vi "RTM Add a new channel.vi"(8 "error in (no error)":errorcluster, 11 "Node Ptr":u64 format="%.0x") -> (0 "error out":errorcluster)   [LabVIEW 2016, in "Async UDP System Explorer.lvlib"]
uses:
  System Explorer/Async UDP System Explorer.lvlib
  <vilib>/NI Veristand/Custom Device API/Custom Device Channel.ctl
  <vilib>/NI Veristand/Custom Device API/Custom Device Channel Type.ctl
  <vilib>/NI Veristand/Custom Device API/Custom Device API.lvlib
panel:
  in  "Tag":string
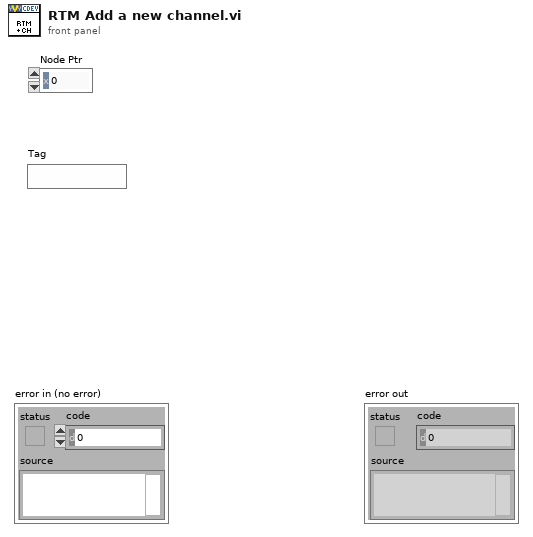
[diagram p1: front panel]
types:
  T1 = typedef "Custom Device API.lvlib/Custom Device Channel.ctl" = cluster{"Type":T2, "Units":string, "Default Value":dbl, "Faultable":bool, "Scalable":bool}
  T2 = typedef "Custom Device API.lvlib/Custom Device Channel Type.ctl" = enum16{"Input", "Output"}
  T3 = typedef "Custom Device API.lvlib/Custom Device Item Ref.ctl" = u64
  T4 = typedef "Custom Device API.lvlib/Custom Device Item Info.ctl" = cluster{"Name":string, "Is Channel":bool, "GUID":string, "Is Waveform":bool}
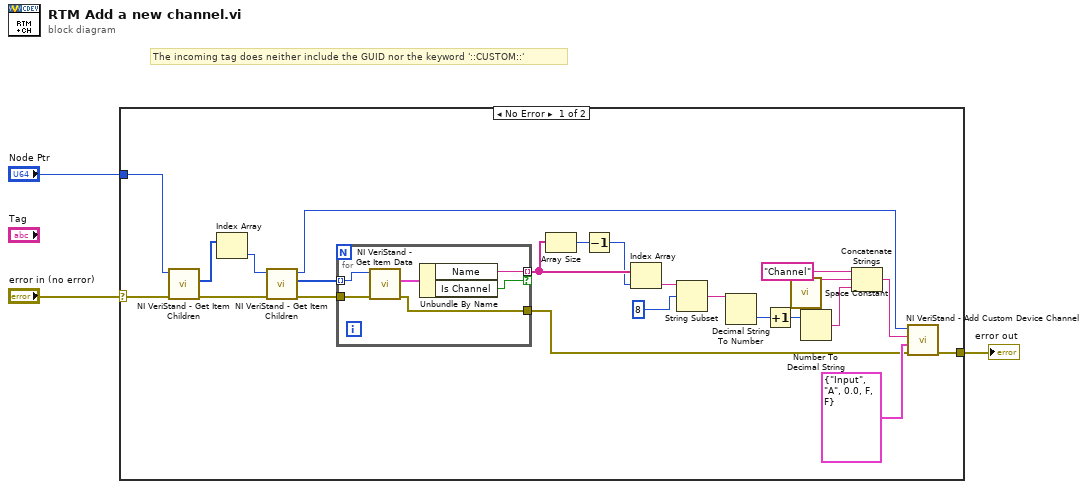
[diagram p0: block diagram]
diagram:
  # "The incoming tag does neither include the GUID nor the keyword '::CUSTOM::'"
  n1 = case shown="No Error" "error in (no error)" {
    selector: "error in (no error)" -> [w26 w33]
    tunnel: "Node Ptr" -> [w25 _]
    tunnel: [w4 w33] -> w1
    frame No Error {
      n2 = call <vilib>:"NI VeriStand - Get Item Children.vi"("error in (no error)"=w26, "Item Ref in"=w25) -> ("error out"=w22:errorcluster, "Child Refs"=w24:T3[])  [unwired: 6 in, 2 out]
      n3 = Index Array(array=w24) -> (element=w23:T3)  [unwired: 1 in]
      n4 = call <vilib>:"NI VeriStand - Get Item Children.vi"("error in (no error)"=w22, "Item Ref in"=w23) -> ("error out"=w21:errorcluster, "Child Refs"=w20:T3[], "Item Ref out"=w10:T3)  [unwired: 6 in, 1 out]
      n5 = for {
        tunnel: w21 -> [w32]
        tunnel: w20 -> [w31] mode=indexing
        tunnel: [w29] -> w18 mode=indexing if=w28
        tunnel: [w27] -> w11
        n6 = call <vilib>:"NI VeriStand - Get Item Data.vi"("error in (no error)"=w32, "Item Ref in"=w31) -> ("error out"=w27:errorcluster, "Item Info"=w30:T4)  [unwired: 6 in, 2 out]
        n7 = Unbundle By Name(w30) -> ("Name"=w29:string, "Is Channel"=w28:bool)
      }
      n8 = Array Size(array=w18) -> (size(s)=w19:i32)
      n9 = Decrement(x=w19) -> (x-1=w17:i32)
      n10 = Index Array(array=w18, index=w17) -> (element=w16:string)
      n11 = String Subset(string=w16, offset (0)=8) -> (substring=w14:string)  [unwired: 1 in]
      n12 = Decimal String To Number(string=w14) -> (number=w13:i32)  [unwired: 2 in, 1 out]
      n13 = Increment(x=w13) -> (x+1=w7:i32)
      n14 = call <vilib>:"Space Constant.vi"() -> ("String"=w8:string)
      n15 = Number To Decimal String(number=w7) -> (decimal integer string=w6:string)  [unwired: 1 in]
      n16 = Concatenate Strings("Channel", w8, w6) -> (w5:string)
      n17 = call <vilib>:"NI VeriStand - Add Custom Device Channel.vi"("error in (no error)"=w11, "Channel"=T1 {"Type"=enum."Input", "Units"="A", "Default Value"=0.0, "Faultable"=FALSE, "Scalable"=FALSE}, "Channel Name"=w5, "Parent Ref in"=w10) -> ("error out"=w4:errorcluster)  [unwired: 4 in, 3 out]
    }
    frame Error {
    }
  }
  "error out" <- w1
